vi "ChangeGraphRefV2.vi"(8 "error in (no error)":errorcluster caption="entrée d'erreur (pas d'erreur)", 9 "CurvesIndx":i32[](array[numeric]), 10 "NewGraphIndex":i32, 11 "Interface en entrée":refnum<class "Interface.lvclass"> caption="DNL_LabVIEW Object in") -> (0 "error out":errorcluster caption="sortie d'erreur", 3 "Interface en sortie":refnum<class "Interface.lvclass"> caption="DNL_LabVIEW Object out")   [LabVIEW 2012, in "Interface.lvclass"]
uses:
  Interface.lvclass
  Interface.lvclass/Interface.ctl
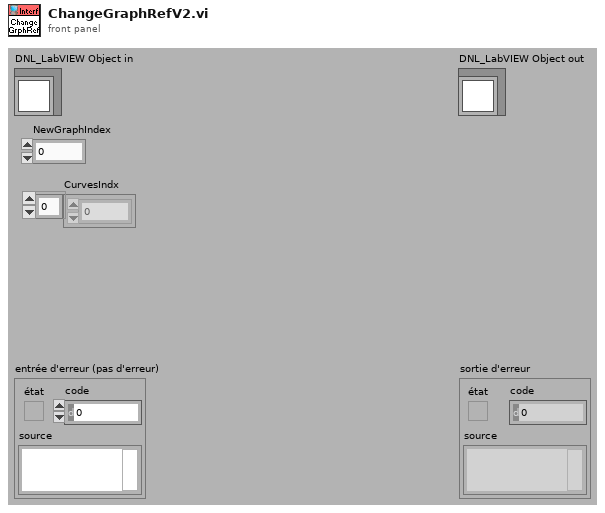
[diagram p1: front panel]
types:
  T1 = typedef "Interface.lvclass/CurveSetup.ctl" = cluster{"CurveName":string, "YParam":string, "XParam":string, "ZParam ":string, "GroupName":string, "LinWdth":u8, "PntCol":u32, "LinCol":u32, "LablFor":u8, "XScale":u32, "YScale":u32, "Interpol":u8, "DisplayName":string, "FillType":i16, "LineStyle":u8, "PntStyle":u8, "BarTyp":u8, "GraphIndex":i32, "Visible":bool, "XScaleName":string, "YScaleName":string, "XYGraph_Ref":refnum<vi>, "Data Only":bool, "DataQ Ref":refnum<queue>, "XParQ Ref":refnum<queue>, "XParamInd":i32, "ScanInd":i32}
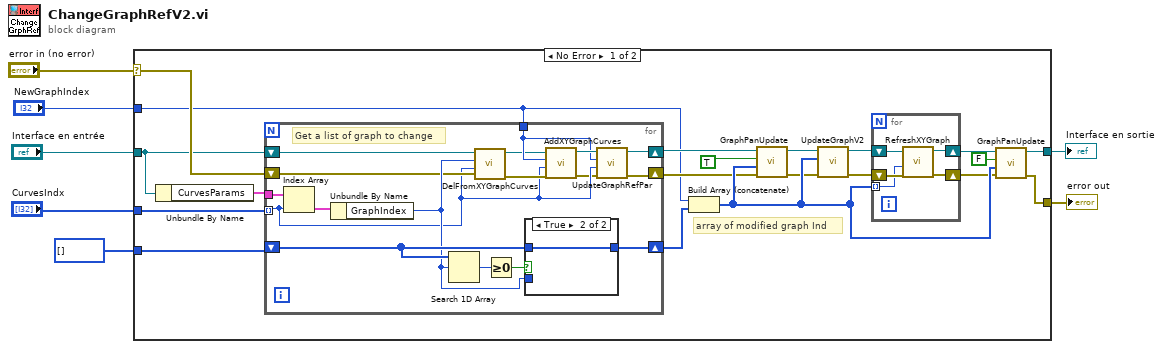
[diagram p0: block diagram]
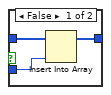
[diagram p2: hidden frame]
diagram:
  n1 = case shown="No Error" "error in (no error)" {
    selector: "error in (no error)" -> [w15 w55]
    tunnel: [w12 w55] -> w6
    tunnel: [w13 w54] -> w4
    tunnel: "Interface en entrée" -> [w8 w54]
    tunnel: "CurvesIndx" -> [w11 _]
    tunnel: "NewGraphIndex" -> [w14 _]
    tunnel: i32[] [] -> [w10 _]
    frame No Error {
      # "array of modified graph Ind"
      n2 = Unbundle By Name(w8) -> ("CurvesParams"=w9:T1[])
      n3 = for {
        tunnel: w9 -> [w44]
        tunnel: w11 -> [w32] mode=indexing
        shift-right: [w40] -> w26
        shift-left: w10 -> [w39]
        shift-right: [w29] -> w20
        shift-left: w8 -> [w37]
        shift-right: [w30] -> w19
        shift-left: w15 -> [w36]
        tunnel: w14 -> [w33]
        # "Get a list of graph to change"
        n4 = Index Array(array=w44, index=w32) -> (element=w43:T1)
        n5 = Unbundle By Name(w43) -> ("GraphIndex"=w38:i32)
        n6 = Search 1D Array(1D array=w39, element=w38) -> (index of element=w41:i32)  [unwired: 1 in]
        n7 = call "DelFromXYGraphCurves.vi"("error in (no error)"=w36, "CurvIndex"=w32, "GraphIndex"=w38, "Interface en entrée"=w37) -> ("error out"=w35:errorcluster, "Interface en sortie"=w28:refnum<class "Interface.lvclass">)  [unwired: 6 in]
        n8 = Greater Or Equal To 0?(x=w41) -> (x >= 0?=w42:bool)
        n9 = case shown="True" w42 {
          tunnel: w39 -> [w47 w48]
          tunnel: [w45 w48] -> w40
          tunnel: w38 -> [w46 _]
          frame False {
            n10 = Insert Into Array(array=w47, new element=w46) -> (w45:i32[])  [unwired: 1 in]
          }
          frame True {
          }
        }
        n11 = call "AddXYGraphCurves.vi"("error in (no error)"=w35, "CurvIndex"=w32, "GraphIndex"=w33, "Interface en entrée"=w28) -> ("error out"=w31:errorcluster, "Interface en sortie"=w34:refnum<class "Interface.lvclass">)  [unwired: 6 in]
        n12 = call "UpdateGraphRefPar.vi"("error in (no error)"=w31, "CurvIndex"=w32, "NewGraphIndex"=w33, "Interface en entrée"=w34) -> ("error out"=w30:errorcluster, "Interface en sortie"=w29:refnum<class "Interface.lvclass">)  [unwired: 5 in, 1 out]
      }
      n13 = Build Array (concatenate)(w14, w26) -> (w27:i32[])
      n14 = call "GraphPanUpdate.vi"("error in (no error)"=w19, "GraphInd"=w27, "DeferUpdate"=TRUE, "Interface en entrée"=w20) -> ("error out"=w22:errorcluster, "Interface en sortie"=w21:refnum<class "Interface.lvclass">)  [unwired: 6 in]
      n15 = call "UpdateGraphV2.vi"("error in (no error)"=w22, "GraphIndexArr"=w27, "Interface en entrée"=w21) -> ("error out"=w23:errorcluster, "Interface en sortie"=w24:refnum<class "Interface.lvclass">)  [unwired: 7 in]
      n16 = for {
        shift-right: [w52] -> w17
        shift-left: w24 -> [w53]
        shift-right: [w50] -> w16
        shift-left: w23 -> [w51]
        tunnel: w27 -> [w49] mode=indexing
        n17 = call "RefreshXYGraph.vi"("error in (no error)"=w51, "Graph Index"=w49, "Interface en entrée"=w53) -> ("error out"=w50:errorcluster, "Interface en sortie"=w52:refnum<class "Interface.lvclass">)  [unwired: 6 in, 1 out]
      }
      n18 = call "GraphPanUpdate.vi"("error in (no error)"=w16, "GraphInd"=w27, "DeferUpdate"=FALSE, "Interface en entrée"=w17) -> ("error out"=w12:errorcluster, "Interface en sortie"=w13:refnum<class "Interface.lvclass">)  [unwired: 6 in]
    }
    frame Error {
    }
  }
  "error out" <- w6
  "Interface en sortie" <- w4
